vi "Write to File Shift Target Information.vi"(4 "Actual Per hour":u32, 5 "Target Cummulative Per Hour":u32, 6 "Target Cummulative Per Shift":u32, 7 "Shift":string, 8 "error in":errorcluster, 9 "Taregt Per Shift":u32, 10 "FTT Percentage":u32, 11 "Refnum in":T1) -> (0 "error out":errorcluster, 3 "refnum out":T1)   [LabVIEW 2018]
uses:
  <vilib>/Utility/config.llb/Config Data RefNum.ctl
  <vilib>/Utility/config.llb/Write Key (U32).vi
  <vilib>/Utility/config.llb/NI_LVConfig.lvlib
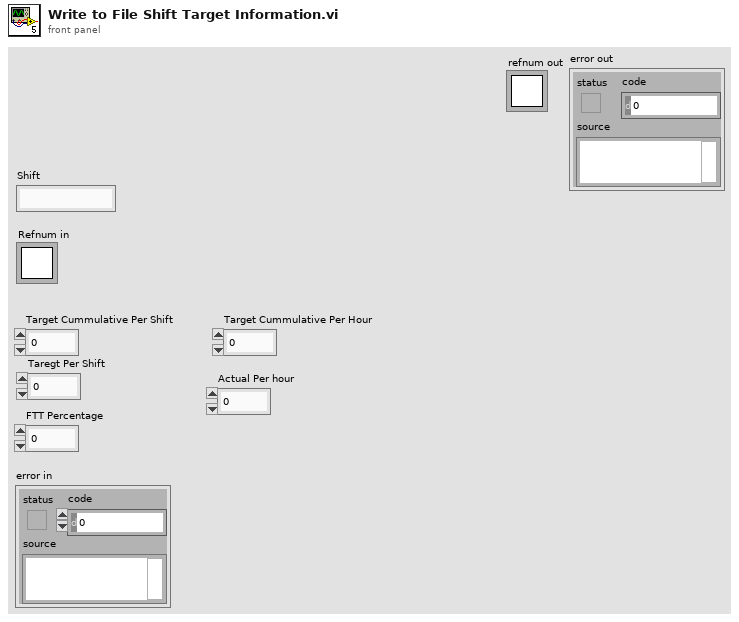
[diagram p1: front panel]
types:
  T1 = typedef "NI_LVConfig.lvlib/Config Data RefNum.ctl" = refnum<k1>
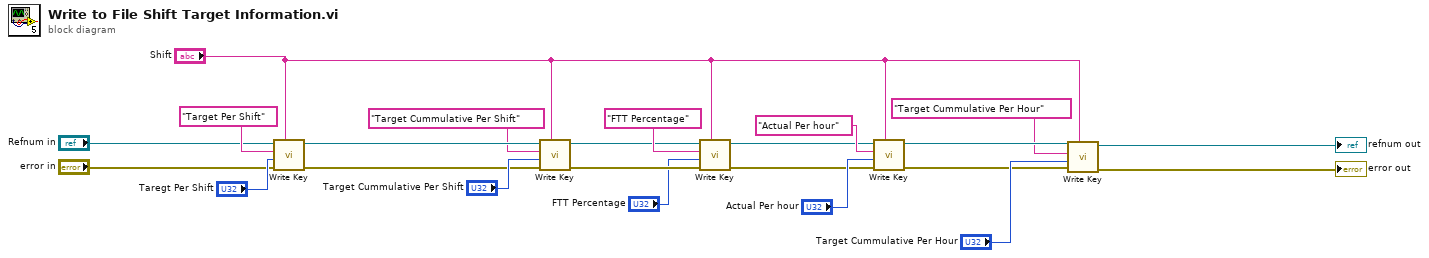
[diagram p0: block diagram]
diagram:
  n1 = call-poly <vilib>:"Write Key.vi"("section"="Shift", "error in (no error)"="error in", "value"="Taregt Per Shift", "key"="Target Per Shift", "refnum"="Refnum in") -> ("error out"=w22:errorcluster, "refnum out"=w21:T1)  [unwired: 4 in, 1 out]
  n2 = call-poly <vilib>:"Write Key.vi"("section"="Shift", "error in (no error)"=w22, "value"="Target Cummulative Per Shift", "key"="Target Cummulative Per Shift", "refnum"=w21) -> ("error out"=w14:errorcluster, "refnum out"=w13:T1)  [unwired: 4 in, 1 out]
  n3 = call-poly <vilib>:"Write Key.vi"("section"="Shift", "error in (no error)"=w14, "value"="FTT Percentage", "key"="FTT Percentage", "refnum"=w13) -> ("error out"=w6:errorcluster, "refnum out"=w7:T1)  [unwired: 4 in, 1 out]
  n4 = call-poly <vilib>:"Write Key.vi"("section"="Shift", "error in (no error)"=w6, "value"="Actual Per hour", "key"="Actual Per hour", "refnum"=w7) -> ("error out"=w5:errorcluster, "refnum out"=w4:T1)  [unwired: 4 in, 1 out]
  n5 = call-poly <vilib>:"Write Key.vi"("section"="Shift", "error in (no error)"=w5, "value"="Target Cummulative Per Hour", "key"="Target Cummulative Per Hour", "refnum"=w4) -> ("error out"=→"error out":errorcluster, "refnum out"=→"refnum out":T1)  [unwired: 4 in, 1 out]
